vi "DFD Filter Response.vi"(10 "IIR Filter Cluster":T1, 11 "fs (Hz)":dbl) -> (2 "ENBW (Hz)":dbl, 3 "XY Graph":cluster{"Ramp Pattern":dbl[], "magnitude":dbl[]}(graph))   [LabVIEW 2019]
uses:
  <vilib>/Analysis/1siggen.llb/Ramp Pattern by Samples.vi
  <vilib>/addons/Digital Filter Design/NI_DigFilterLicensed.lvlib
  <vilib>/Analysis/NI_AALBase.lvlib
  <vilib>/Analysis/NI_AALPro.lvlib
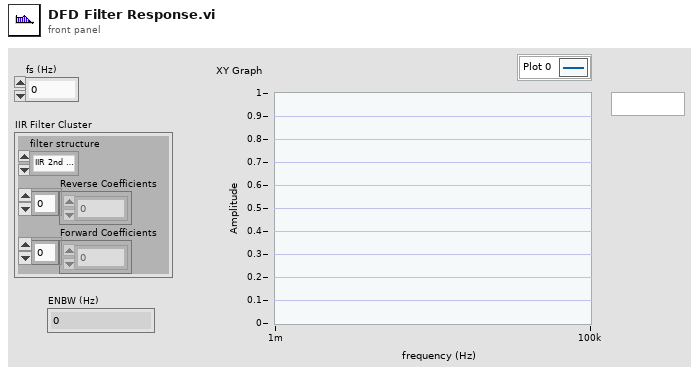
[diagram p1: front panel]
types:
  T1 = cluster{"filter structure":enum32{"IIR 2nd Order", "IIR 4th Order"}, "Reverse Coefficients":dbl[], "Forward Coefficients":dbl[]}
  T2 = typedef "NI_DigFilterLicensed.lvlib/DFD Filter Obj.ctl" = cluster{"mSRate_Fs":dbl, "mSRate_Version":string, "mSRate_Comments":string, "mSRate_OrgCoef":T3, "mSRate_CurCoef":T3, "mSRate_Quantized?":bool, "mSRate_QCoef":T3, "mSRate_QSettings":T5[], "mSRate_Order":i32, "mSRate_Scaling":cluster{"mSRate_ScaleByPowerOf2?":bool, "mSRate_ScaleType":T7}}
  T3 = typedef "NI_DigFilterLicensed.lvlib/DFD Filter Coef.ctl" = cluster{"type":T4, "gain":dbl, "coef a (k)":dbl[], "coef b (v)":dbl[]}
  T4 = typedef "NI_DigFilterLicensed.lvlib/DFD Filter Structure Type Selector.ctl" = enum16{"Undefined", "FIR Direct Form", "FIR Direct Form Transposed", "FIR Symmetric", "FIR Antisymmetric", "IIR Direct Form I", "IIR Direct Form I Transposed", "IIR Direct Form II", "IIR Direct Form II Transposed", "IIR Cascaded Second Order Sections Form I", "IIR Cascaded Second Order Sections Form I Transposed", "IIR Cascaded Second Order Sections Form II", "IIR Cascaded Second Order Sections Form II Transposed", "Lattice Allpass (basic sections)", "Lattice Allpass (one multiplier sections)", "Lattice Allpass (normalized sections)", "Lattice AR (basic sections)", "Lattice AR (one multiplier sections)", "Lattice AR (normalized sections)", "Lattice MA (minimum phase)", "Lattice MA (maximum phase)", "Lattice ARMA (basic sections)", "Lattice ARMA (one multiplier sections)", "Lattice ARMA (normalized sections)"}
  T5 = typedef "NI_DigFilterLicensed.lvlib/dfd_Internal Quantization Settings.ctl" = cluster{"source":T6, "wl":i16, "iwl":i16, "overflow mode":enum16{"Saturation", "Wrap"}, "rounding mode":enum16{"Nearest", "Truncation"}, "signed?":bool}
  T6 = typedef "NI_DigFilterLicensed.lvlib/dfd_Internal Quantization Srcs.ctl" = u16
  T7 = typedef "NI_DigFilterLicensed.lvlib/DFD Coef Norm Type.ctl" = enum16{"No Norm", "Time Domain 1-Norm", "Time Domain 2-Norm", "Time Domain Inf-Norm"}
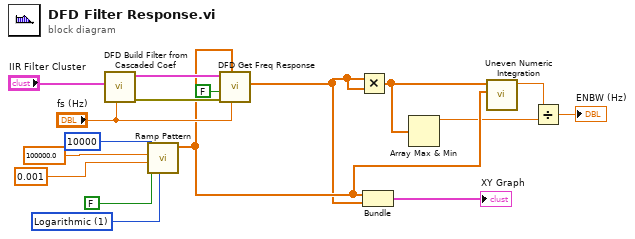
[diagram p0: block diagram]
diagram:
  w10 = u16 1 items=["Linear", "Logarithmic"] ("type")
  n1 = call <vilib>:"DFD Build Filter from Cascaded Coef.vi"("fs [Hz]"="fs (Hz)", "IIR Filter Cluster"="IIR Filter Cluster") -> ("error out"=w16:errorcluster, "filter out"=w9:T2)  [unwired: 8 in]
  n2 = call-poly <vilib>:"Ramp Pattern.vi"("type"=w10, "exclude end?"=FALSE, "start"=0.001, "end"=100000.0, "samples"=10000) -> ("Ramp Pattern"=w6:dbl[])  [unwired: 5 in, 1 out]
  n3 = call <vilib>:"DFD Get Freq Response.vi"("fs [Hz]"="fs (Hz)", "freq points [Hz]"=w6, "error in (no error)"=w16, "dB on? (T)"=FALSE, "filter in"=w9) -> ("magnitude"=w1:dbl[])  [unwired: 3 in, 3 out]
  n4 = Multiply(x=w1, y=w1) -> (x*y=w5:dbl[])
  n5 = Bundle("Ramp Pattern"=w6, "magnitude"=w1) -> (→"XY Graph":cluster{"Ramp Pattern":dbl[], "magnitude":dbl[]})  [unwired: 1 in]
  n6 = Array Max & Min(array=w5) -> (max value=w3:dbl)  [unwired: 3 out]
  n7 = call <vilib>:"Uneven Numeric Integration.vi"("T"=w6, "X"=w5) -> ("result"=w4:dbl)  [unwired: 8 in, 1 out]
  n8 = Divide(x=w4, y=w3) -> (x/y=→"ENBW (Hz)":dbl)
